vi "Delete Data sub_ UT.vi"(8 "error in (no error)":errorcluster, 10 "No. of Rows":i64, 11 "TableLogger_SQLite_Actor in":refnum<class "TableLogger_SQLite_Actor.lvclass">) -> (0 "error out":errorcluster, 2 "Deleted?T":bool, 3 "TableLogger_SQLite_Actor out":refnum<class "TableLogger_SQLite_Actor.lvclass">)   [LabVIEW 2014, in "TableLogger_SQLite_Actor.lvlib" / "TableLogger_SQLite_Actor.lvclass"]
uses:
  TableLogger_SQLite_Actor.lvclass
  TableLogger_SQLite_Actor.lvclass/TableLogger_SQLite_Actor.ctl
  <vilib>/drjdpowell/SQLite Library/SQL Connection/Execute SQL (Single Integer).vi
  <vilib>/drjdpowell/SQLite Library/SQLite.lvlib
  <vilib>/drjdpowell/SQLite Library/SQL Connection/Connection.lvclass
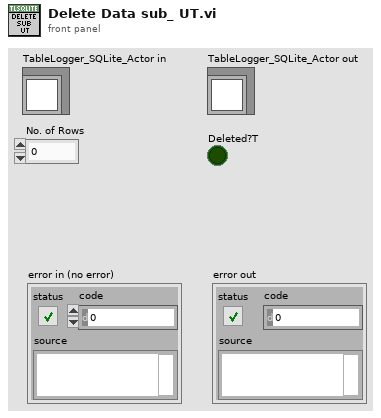
[diagram p1: front panel]
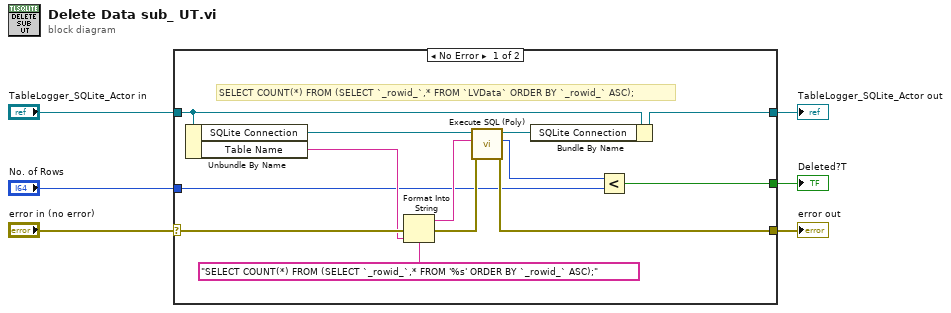
[diagram p0: block diagram]
diagram:
  n1 = case shown="No Error" "error in (no error)" {
    selector: "error in (no error)" -> [w15 w21]
    tunnel: [w19 w20] -> w6
    tunnel: "TableLogger_SQLite_Actor in" -> [w18 w20]
    tunnel: [w9 _] -> w3
    tunnel: [w14 w21] -> w2
    tunnel: "No. of Rows" -> [w7 _]
    frame No Error {
      # "SELECT COUNT(*) FROM (SELECT `_rowid_`,* FROM `LVData` ORDER BY `_rowid_` ASC);"
      n2 = Unbundle By Name(w18) -> ("SQLite Connection"=w13:refnum<class "Connection.lvclass">, "Table Name"=w8:string)
      n3 = Format Into String(format string="SELECT COUNT(*) FROM (SELECT `_rowid_`,* FROM '%s' ORDER BY `_rowid_` ASC);" ("SQL"), error in=w15, w8) -> (resulting string=w11:string, error out=w16:errorcluster)  [unwired: 1 in]
      n4 = call-poly <vilib>:"Execute SQL (Poly).vi"("error in (no error)"=w16, "SQL"=w11, "SQLite Connection in"=w13) -> ("error out"=w14:errorcluster, "Result"=w10:i64, "SQLite Connection"=w17:refnum<class "Connection.lvclass">)  [unwired: 6 in]
      n5 = Bundle By Name(cluster=w18, "SQLite Connection"=w17) -> (w19:refnum<class "TableLogger_SQLite_Actor.lvclass">)
      n6 = Less?(x=w10, y=w7) -> (x < y?=w9:bool)
    }
    frame Error {
    }
  }
  "Deleted?T" <- w3
  "TableLogger_SQLite_Actor out" <- w6
  "error out" <- w2
